vi "Actor Core.vi"(8 "error in":errorcluster, 11 "PLC Sim Controller Actor in":refnum<class "PLC Sim Controller Actor.lvclass">) -> (0 "error out":errorcluster, 3 "Actor out":refnum<class "Actor.lvclass">)   [LabVIEW 2019, in "PLC Sim Controller Actor.lvlib" / "PLC Sim Controller Actor.lvclass"]
doc: "(<B>Filename</B>: Actor Framework.lvlib:Actor.lvclass:Actor Core.vi)\n\nReceives messages to the actor, reacts to them, and initiates any error handling that may shut the actor down.\n\nDescendant classes may override this VI to append parallel tasks for the actor to complete while it handles messages. Overrides use the Call Parent Method node."
uses:
  PLC Sim Controller Actor.lvclass
  C:/Program Files (x86)/National Instruments/LabVIEW 2019/vi.lib/ActorFramework/Actor/Actor.lvclass
  <vilib>/ActorFramework/Actor/Actor.lvclass
  <vilib>/Utility/miscctls.llb/LVComboBoxStrsAndValuesArrayTypeDef.ctl
  PLC Sim Controller Actor.lvclass/PLC Sim Controller Actor.ctl
  <vilib>/ActorFramework/Actor/Actor.lvclass/Actor.ctl
  <vilib>/ActorFramework/Message Enqueuer/Message Enqueuer.lvclass/Message Enqueuer.ctl
  PLC Sim Controller Actor Messages/Select Station Msg/Select Station Msg.lvclass/Select Station Msg.ctl
  <vilib>/ActorFramework/Message Enqueuer/Init from Existing Queue.vi
  <vilib>/ActorFramework/Message Enqueuer/Enqueue.vi
  PLC Sim Controller Actor Messages/Enable Create Station Msg/Enable Create Station Msg.lvclass
  C:/Program Files (x86)/National Instruments/LabVIEW 2019/vi.lib/ActorFramework/Message/Message.lvclass
  <vilib>/ActorFramework/Stop Msg/Stop Msg.lvclass
  PLC Sim Controller Actor Messages/Create Station Msg/Create Station Msg.lvclass
  PLC Sim Controller Actor Messages/Select Station Msg/Select Station Msg.lvclass
  <vilib>/ActorFramework/Message Priority Queue/Priority Enqueue.vi
  <vilib>/ActorFramework/Message Enqueuer/Message Enqueuer.lvclass
panel:
  out "Pause/Resume":bool
  in  "Online Stations":string(combo)
  in  "Create Station":bool
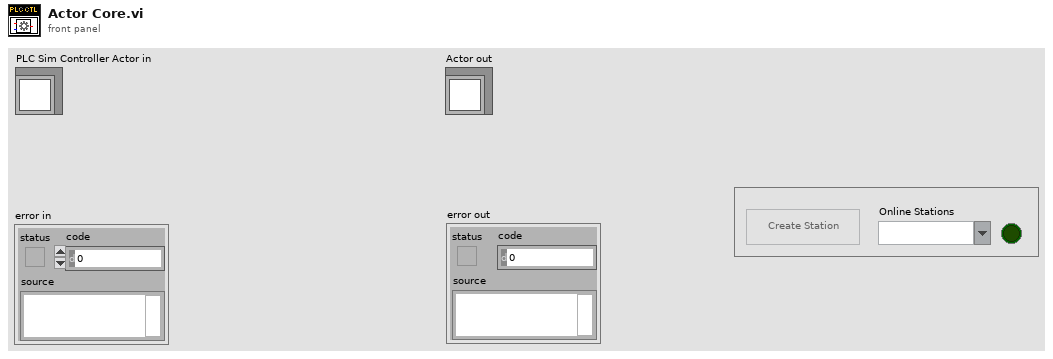
[diagram p1: front panel]
types:
  T1 = typedef "LVComboBoxStrsAndValuesArrayTypeDef.ctl" = cluster{"String":string, "Value":string}[]
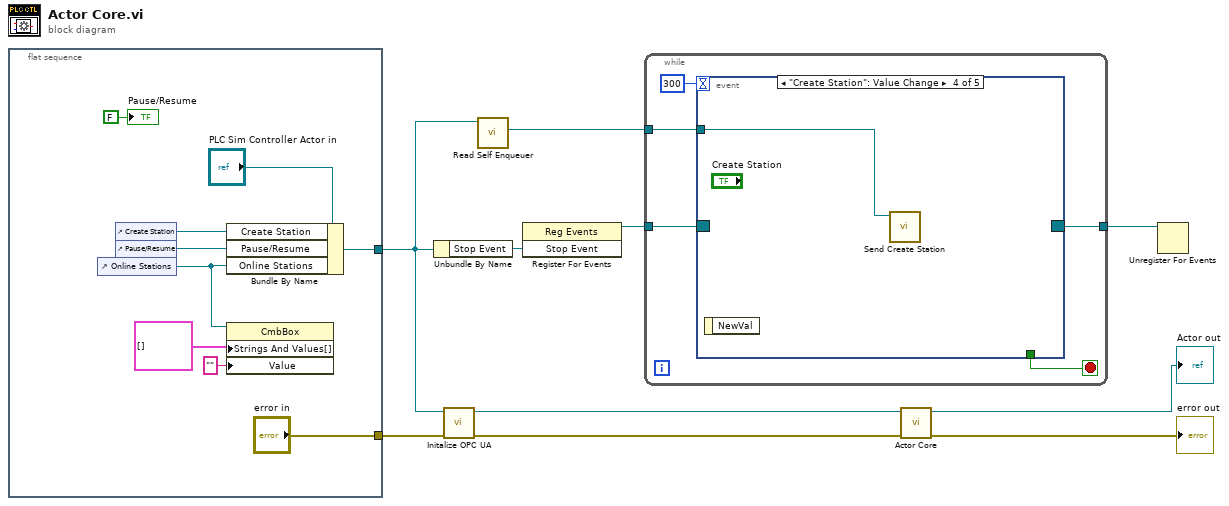
[diagram p0: block diagram]
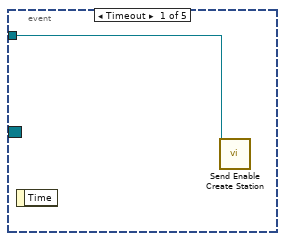
[diagram p2: hidden frame]
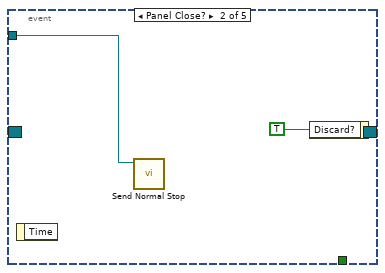
[diagram p3: hidden frame]
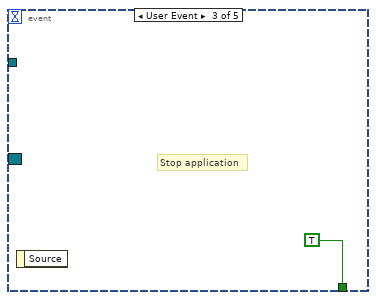
[diagram p4: hidden frame]
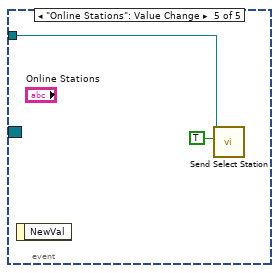
[diagram p5: hidden frame]
diagram:
  n1 = flat-sequence {
    tunnel: ["error in"] -> w2
    tunnel: [w16] -> w4
    frame #0 {
      n2 = control-ref of="Online Stations"() -> (w13:refnum<vi>)
      n3 = control-ref of="Create Station"() -> (w17:refnum<vi>)
      n4 = control-ref of="Pause/Resume"() -> (w15:refnum<vi>)
      n5 = Bundle By Name(cluster="PLC Sim Controller Actor in", "Create Station"=w17, "Pause/Resume"=w15, "Online Stations"=w13) -> (w16:refnum<class "PLC Sim Controller Actor.lvclass">)
      n6 = property class="CmbBox"(reference=w13, "Strings And Values[]"=T1 [] ("Strings And Values []"), "Value"="") -> ()  [unwired: 1 in, 2 out]
      "Pause/Resume" <- FALSE ("Pause/Resume")
    }
  }
  n7 = Unbundle By Name(w4) -> ("Stop Event"=w8:refnum<user-event>)
  n8 = call "Initalize OPC UA.vi"("error in (no error)"=w2, "SM EOL Station Actor in"=w4) -> ("error out"=w1:errorcluster, "SM EOL Station Actor out"=w3:refnum<class "PLC Sim Controller Actor.lvclass">)  [unwired: 8 in]
  n9 = call <vilib>:"Read Self Enqueuer.vi"("Actor"=w4) -> ("Self Enqueuer"=w5:refnum<class "Message Enqueuer.lvclass">)  [unwired: 10 in]
  n10 = register-events(w8) -> (reference out=w7:refnum<event-registration>)  [unwired: 2 in, 1 out]
  n11 = while {
    tunnel: w7 -> [w23]
    tunnel: [w22] -> w6
    tunnel: w5 -> [w21]
    stop <- w24 stop-if-true
    n12 = event shown="[3] \"Create Station\": Value Change" {
      selector: w23 -> [_ _ _ _ _]
      dyn-events: [_ _ _ _ _] -> w22
      timeout: 300 -> [_ _ _ _ _]
      tunnel: [_ _ TRUE _ _] -> w24
      tunnel: w21 -> [w25 w26 _ w29 w31]
      event Timeout {
        n13 = event-data() -> ()  [unwired: 1 in, 1 out]
        n14 = call "Send Enable Create Station.vi"("Message Enqueuer"=w25) -> ()  [unwired: 9 in, 2 out]
      }
      event Panel Close? {
        n15 = event-data() -> ()  [unwired: 1 in, 1 out]
        n16 = call <vilib>:"Send Normal Stop.vi"("Message Enqueuer"=w26) -> ()  [unwired: 10 in, 1 out]
        n17 = event-data("Discard?"=TRUE) -> ()  [unwired: 1 in, 1 out]
      }
      event User Event {
        # "Stop application"
        n18 = event-data() -> ()  [unwired: 1 in, 1 out]
      }
      event "Create Station": Value Change {
        n19 = event-data() -> ()  [unwired: 1 in, 1 out]
        n20 = call "Send Create Station.vi"("Message Enqueuer"=w29) -> ()  [unwired: 9 in, 2 out]
      }
      event "Online Stations": Value Change {
        n21 = event-data() -> ()  [unwired: 1 in, 1 out]
        n22 = call "Send Select Station.vi"("FP Frontmost"=TRUE, "Message Enqueuer"=w31) -> ()  [unwired: 8 in, 2 out]
      }
    }
  }
  n23 = call-parent "Actor Core.vi"("error in"=w1, "Actor in"=w3) -> ("error out"=→"error out":errorcluster, "Actor out"=→"Actor out":refnum<class "Actor.lvclass">)  [unwired: 8 in]
  n24 = Unregister For Events(event registration refnum=w6) -> ()  [unwired: 1 in, 1 out]
